vi "Test_MCP_Server.vi"(8 "error in (no error)":errorcluster) -> (0 "error out":errorcluster)   [LabVIEW 2020, in "MCP Server tests.lvlib"]
uses:
  MCP Server tests.lvlib
  416cc145-bc65-4336-831b-dce381f7377e.vi
  fake tool add.vi
  fake_tool_say_hello.vi
  fake tool return error.vi
  fake tool broken vi.vi
  fake tool no inputs outputs.vi
  fake tool ignored.vi
  fake resource short string.vi
  fake resource long string.vi
  fake resource broken vi.vi
  fake prompt broken vi.vi
  fake prompt concatanate strings.vi
  fake tool no description.vi
  src/MCP Server/MCP Server.lvlib
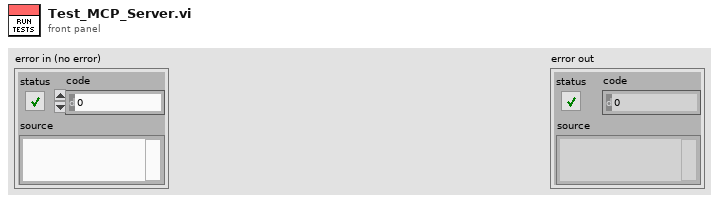
[diagram p1: front panel]
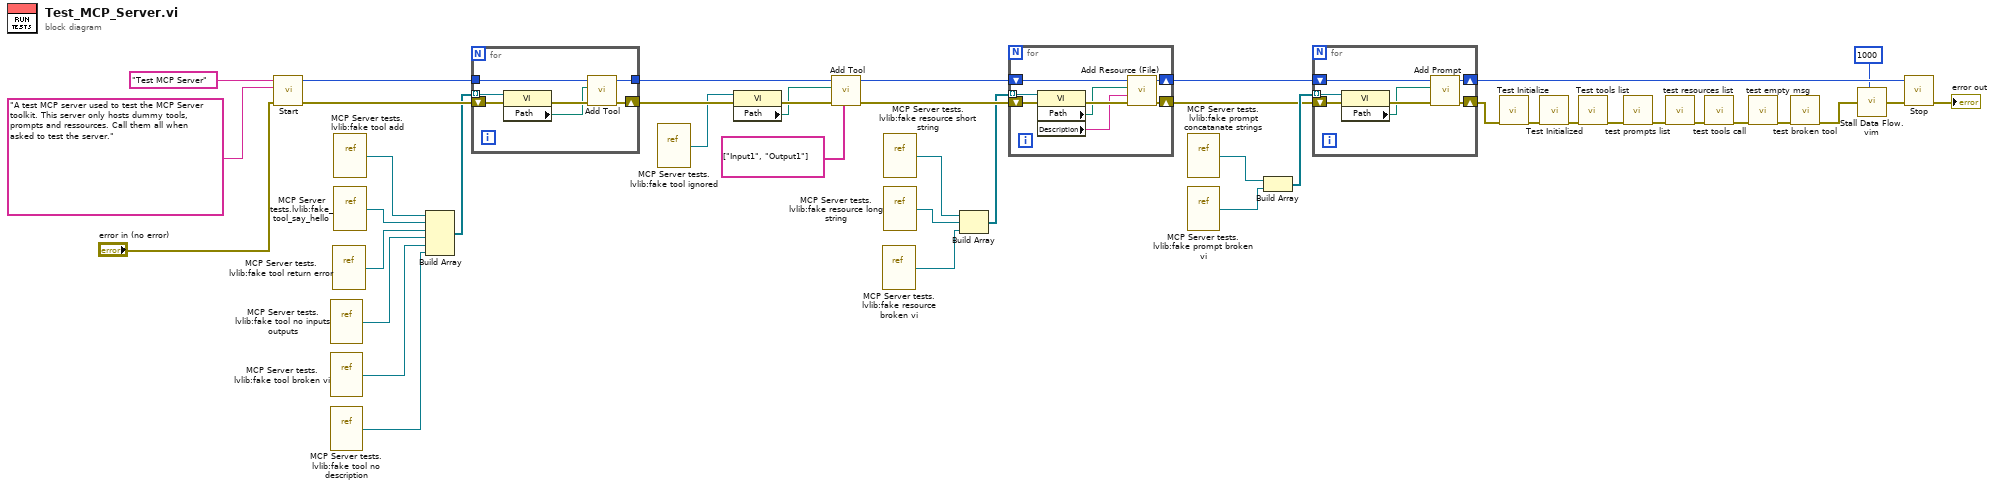
[diagram p0: block diagram]
diagram:
  n1 = call "Start.vi"("error in (no error)"="error in (no error)", "Description"="A test MCP server used to test the MCP Server toolkit. This server only hosts dummy tools, prompts and ressources. Call them all when asked to test the server.", "Name"="Test MCP Server") -> ("error out"=w42:errorcluster, "server id out"=w35:i32)  [unwired: 6 in, 1 out]
  n2 = vi-ref "MCP Server tests.lvlib:fake tool no inputs outputs.vi"() -> (w16:refnum<vi>)
  n3 = vi-ref "MCP Server tests.lvlib:fake tool broken vi.vi"() -> (w7:refnum<vi>)
  n4 = vi-ref "MCP Server tests.lvlib:fake tool no description.vi"() -> (w3:refnum<vi>)
  n5 = vi-ref "MCP Server tests.lvlib:fake tool return error.vi"() -> (w37:refnum<vi>)
  n6 = vi-ref "MCP Server tests.lvlib:fake tool add.vi"() -> (w39:refnum<vi>)
  n7 = vi-ref "MCP Server tests.lvlib:fake_tool_say_hello.vi"() -> (w38:refnum<vi>)
  n8 = Build Array(w39, w38, w37, w16, w7, w3) -> (w36:refnum<vi>[])
  n9 = for {
    shift-right: [w44] -> w34
    shift-left: w42 -> [w49]
    tunnel: w36 -> [w48] mode=indexing
    tunnel: w35 -> [w46]
    tunnel: [w45] -> w32
    n10 = property class="VI"(reference=w48, error in=w49) -> (error out=w47:errorcluster, "Path"=w43:path)  [unwired: 1 out]
    n11 = call "Add Tool.vi"("error in (no error)"=w47, "vi path"=w43, "server id"=w46) -> ("error out"=w44:errorcluster, "server id out"=w45:i32)  [unwired: 7 in]
  }
  n12 = vi-ref "MCP Server tests.lvlib:fake tool ignored.vi"() -> (w29:refnum<vi>)
  n13 = property class="VI"(reference=w29, error in=w34) -> (error out=w30:errorcluster, "Path"=w28:path)  [unwired: 1 out]
  n14 = call "Add Tool.vi"("Ignored"=string[] ["Input1", "Output1"], "error in (no error)"=w30, "vi path"=w28, "server id"=w32) -> ("error out"=w33:errorcluster, "server id out"=w31:i32)  [unwired: 6 in]
  n15 = vi-ref "MCP Server tests.lvlib:fake resource broken vi.vi"() -> (w2:refnum<vi>)
  n16 = vi-ref "MCP Server tests.lvlib:fake resource short string.vi"() -> (w25:refnum<vi>)
  n17 = vi-ref "MCP Server tests.lvlib:fake resource long string.vi"() -> (w26:refnum<vi>)
  n18 = Build Array(w25, w26, w2) -> (w24:refnum<vi>[])
  n19 = for {
    shift-right: [w56] -> w20
    shift-left: w33 -> [w55]
    shift-right: [w57] -> w21
    shift-left: w31 -> [w54]
    tunnel: w24 -> [w52] mode=indexing
    n20 = property class="VI"(reference=w52, error in=w55) -> (error out=w53:errorcluster, "Path"=w51:path, "Description"=w50:string)  [unwired: 1 out]
    n21 = call "Add Resource (File).vi"("error in (no error)"=w53, "description"=w50, "file path"=w51, "server id"=w54) -> ("error out"=w56:errorcluster, "server id out"=w57:i32)  [unwired: 6 in]
  }
  n22 = vi-ref "MCP Server tests.lvlib:fake prompt concatanate strings.vi"() -> (w22:refnum<vi>)
  n23 = vi-ref "MCP Server tests.lvlib:fake prompt broken vi.vi"() -> (w1:refnum<vi>)
  n24 = Build Array(w22, w1) -> (w23:refnum<vi>[])
  n25 = for {
    shift-right: [w63] -> w18
    shift-left: w20 -> [w62]
    shift-right: [w64] -> w19
    shift-left: w21 -> [w61]
    tunnel: w23 -> [w59] mode=indexing
    n26 = property class="VI"(reference=w59, error in=w62) -> (error out=w60:errorcluster, "Path"=w58:path)  [unwired: 1 out]
    n27 = call "Add Prompt.vi"("error in (no error)"=w60, "vi path"=w58, "server id"=w61) -> ("error out"=w63:errorcluster, "server id out"=w64:i32)  [unwired: 7 in]
  }
  n28 = call "Test Initialize.vi"("error in (no error)"=w18) -> ("error out"=w17:errorcluster)  [unwired: 9 in, 1 out]
  n29 = call "Test Initialized.vi"("error in (no error)"=w17) -> ("error out"=w15:errorcluster)  [unwired: 9 in, 1 out]
  n30 = call "Test tools list.vi"("error in (no error)"=w15) -> ("error out"=w14:errorcluster)  [unwired: 9 in, 1 out]
  n31 = call "test prompts list.vi"("error in (no error)"=w14) -> ("error out"=w13:errorcluster)  [unwired: 9 in, 1 out]
  n32 = call "test resources list.vi"("error in (no error)"=w13) -> ("error out"=w12:errorcluster)  [unwired: 9 in, 1 out]
  n33 = call "test tools call.vi"("error in (no error)"=w12) -> ("error out"=w11:errorcluster)  [unwired: 9 in, 1 out]
  n34 = call "test empty msg.vi"("error in (no error)"=w11) -> ("error out"=w8:errorcluster)  [unwired: 9 in, 1 out]
  n35 = call "test broken tool.vi"("error in (no error)"=w8) -> ("error out"=w6:errorcluster)  [unwired: 9 in, 1 out]
  n36 = call "Stall Data Flow.vim"("value in"=w6, "milliseconds to wait"=u32 1000) -> ("value out"=w5:errorcluster)  [unwired: 1 out]
  n37 = call "Stop.vi"("error in (no error)"=w5, "id"=w19) -> ("error out"=→"error out":errorcluster)  [unwired: 9 in]
